vi "ALL2.vi"() -> ()   [LabVIEW 2016, in "Test2.lvrbt"]
uses:
  Test2.lvrbt
  <vilib>/NXT/Hardware/Plugins/Tetrix DC Motor/TetrixDCMotorAddress.ctl
  <vilib>/NXT/Hardware/Plugins/Tetrix 180 deg Servo/Tetrix180ServoAddress.ctl
  <vilib>/NXT/Block Support/NXT_InputPort.ctl
  <vilib>/NXT/Subs/ColorSensorColors.ctl
  <vilib>/NXT/NXTIO Xnodes/NXTIONodeSubVIs/TETRIX IO Move Servos.vi
  <vilib>/NXT/Dual Mode Library/Waits/Wait_Num.vi
  <vilib>/NXT/NXTIO Xnodes/NXTIONodeSubVIs/TETRIX IO Move DC Motors.vi
  <vilib>/NXT/NXTIO Xnodes/NXTIONodeSubVIs/TETRIX IO Stop DC Motors.vi
  <vilib>/NXT/Dual Mode Library/Waits/Wait_EV3_Ultrasonic_Centimeter_Closer.vi
  <vilib>/NXT/Dual Mode Library/Waits/Wait_EV3_Ultrasonic_Centimeters_Further.vi
  <vilib>/NXT/Dual Mode Library/Waits/Wait_Touch.vi
  <vilib>/NXT/Dual Mode Library/Waits/Wait_EV3_Color_Color.vi
  <vilib>/NXT/Dual Mode Library/Sensors/EV3_Ultrasonic_CM.vi
  <vilib>/NXT/NXTIO Xnodes/AddressXNode/NXTIOAddress.xnode
  <vilib>/NXT/Subs/LVHSConnector.ctl
  <vilib>/NXT/NXTIO Xnodes/NXTIOXNode/NXTIO.xnode
  <vilib>/NXT/LegoClasses/BrickReference/BrickReference.lvclass
panel:
  out "Power 3":bool
  out "X Upper Left  2":u8
  out "X Lower Right  2":u8
  out "Y Lower Right  2":u8
  out "Y Upper Left  2":u8
  out "Count 3":u8
  out "Color 3":u8
  in  "Cluster 3":T1 {"Tracking Mode" items=["Disable Tracking", "Get First Object", "Get n th Object", "Enable Tracking", "Sort Objects  by size", "Sort Objects  by Colors", "Illumination on ", "Illumination Off", "Write Colormap", "Read Colormap", "Line tracking mode", "Object Tracking mode"]}
  out "Power 2":bool
  out "X Upper Left":u8
  out "X Lower Right":u8
  out "Y Lower Right":u8
  out "Y Upper Left":u8
  out "Count 2":u8
  out "Color 2":u8
  in  "Cluster 2":T1 {"Tracking Mode" items=["Disable Tracking", "Get First Object", "Get n th Object", "Enable Tracking", "Sort Objects  by size", "Sort Objects  by Colors", "Illumination on ", "Illumination Off", "Write Colormap", "Read Colormap", "Line tracking mode", "Object Tracking mode"]}
types:
  T1 = cluster{"Address":dbl, "No of Object to track":dbl, "Tracking Mode":u8}
  T2 = typedef "Tetrix180ServoAddress.ctl" = i32
  T3 = cluster{"Tetrix180Servo":T2, "Tetrix180Servo 2":T2, "Tetrix180Servo 3":T2, "Tetrix180Servo 4":T2, "Tetrix180Servo 5":T2, "Tetrix180Servo 6":T2}
  T4 = typedef "TetrixDCMotorAddress.ctl" = i32
  T5 = cluster{"TetrixDCMotor":T4, "TetrixDCMotor 2":T4}
  T6 = cluster{"Tetrix180Servo":T2, "Tetrix180Servo":T2, "Tetrix180Servo":T2, "Tetrix180Servo":T2, "Tetrix180Servo":T2, "Tetrix180Servo":T2}
  T7 = typedef "LVHSConnector.ctl" = refnum<class "BrickReference.lvclass">
  T8 = typedef "NXT_InputPort.ctl" = u32
  T9 = typedef "ColorSensorColors.ctl" = enum16{"No Color", "Black", "Blue", "Green", "Yellow", "Red", "White", "Brown"}
  T10 = cluster{"Tracking Mode":u8, "Object Number to Track":u8, "Address":u8}
  T11 = cluster{"Total Tracked Objects":u8, "Color":u8, "X Upper Left":u8, "Y Upper Left":u8, "X Lower Right":u8, "Y Lower Right":u8, "Status (boolean)":bool}
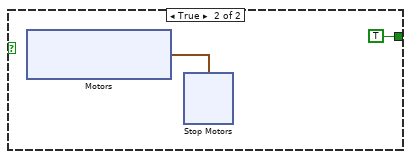
[diagram p2: hidden frame]
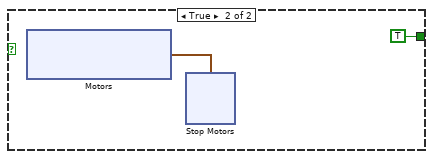
[diagram p3: hidden frame]
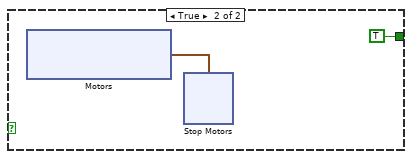
[diagram p4: hidden frame]
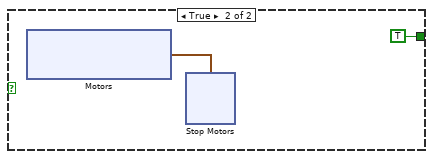
[diagram p5: hidden frame]
diagram:
  # "FILE: BACK TOBASE2\n\nTHE ROBOT WILL GO TO BASE"
  # "FILE: SAVETOUCH \n\nTHE ROBOT WILL DETECT THE RACK \nAND STRAIGHT THE POSITION"
  # "FILE: SAVETOUCH \n\nTHE ROBOT WILL DETECT THE RACK \nAND STRAIGHT THE POSITION"
  # "FILE: DETECT REFERENCE LINE, AFTER AIMING\n\nTHE ROBOT WILL GET A NEW POSITION AFTER LAUNCH THE BALL"
  # "FILE: TRAPBALL\n\nTHE ROBOT WILL MOVE FOWARD TO TRAP THE BALL"
  # "FILE: GETSEECONDBALL\n\nTHE ROBOT WILL START TO DETECT AND PICKUP THE SECOND BALL"
  # "FILE: DETECT REFERENCE LINE, AFTER AIMING\n\nTHE ROBOT WILL GET A NEW POSITION AFTER LAUNCH THE BALL"
  # "FILE: SERVOSETTING\n\nTHE FIRST BALL WILL BE PICKUP"
  # "FILE: DETECTFIRSTBALL\n\nTHE ROBOT WILL MOVE INFRONT TO DETECT THE FIRST BALL"
  # "FILE: SAVETOUCH \n\nTHE ROBOT WILL DETECT THE RACK \nAND STRAIGHT THE POSITION"
  # "FILE:  motor setting\n\nTHE ROBOT WILL MOVE OUT FROM THE BASE."
  n1 = flat-sequence {
    tunnel: [w13] -> w12
    frame #0 {
      n2 = xnode "Motors"() -> ("Motor"=w22:T6)
      n3 = xnode "Move Servos"("Position 6"=u8 28, "Position 5"=u8 237, "Position 4"=u8 40, "Position 3"=u8 7, "Position 2"=u8 0, "Position 1"=u8 220, "Motors"=w22) -> ("NXT/EV3"=w15:T7)  [unwired: 1 in]
      n4 = xnode "Motors"() -> ("Motor"=w27:cluster{"TetrixDCMotor":T4, "TetrixDCMotor":T4})
      n5 = call-poly <vilib>:"PolyWait.vi"("Time (1 sec)"=sgl 1.0, "NXT/EV3"=w15) -> ("NXT/EV3"=w14:T7)  [unwired: 2 in]
      n6 = xnode "Move Motors"("Power/Speed 2"=i8 50, "Power/Speed 1"=i8 50, "Motors"=w27, "NXT/EV3"=w14) -> ("NXT/EV3"=w30:T7)
      n7 = call-poly <vilib>:"PolyWait.vi"("Time (1 sec)"=sgl 2.0, "NXT/EV3"=w30) -> ("NXT/EV3"=w28:T7)  [unwired: 2 in]
      n8 = xnode "Motors"() -> ("Motor"=w33:cluster{"TetrixDCMotor":T4, "TetrixDCMotor":T4})
      n9 = xnode "Stop Motors"("Motors"=w27, "NXT/EV3"=w28) -> ("NXT/EV3"=w26:T7)
      n10 = call-poly <vilib>:"PolyWait.vi"("Time (1 sec)"=sgl 1.0, "NXT/EV3"=w26) -> ("NXT/EV3"=w24:T7)  [unwired: 2 in]
      n11 = xnode "Move Motors"("Power/Speed 2"=i8 50, "Power/Speed 1"=i8 50, "Motors"=w33, "NXT/EV3"=w24) -> ("NXT/EV3"=w36:T7)
      n12 = call-poly <vilib>:"PolyWait.vi"("Time (1 sec)"=sgl 1.5, "NXT/EV3"=w36) -> ("NXT/EV3"=w34:T7)  [unwired: 2 in]
      n13 = xnode "Stop Motors"("Motors"=w33, "NXT/EV3"=w34) -> ("NXT/EV3"=w13:T7)
    }
  }
  n14 = flat-sequence {
    tunnel: w12 -> [w82]
    tunnel: [w81] -> w11
    frame #0 {
      w97 = T8 1 items=["Port 1", "Port 2", "Port 3", "Port 4"] ("Port (Port 1)")
      w113 = T8 1 items=["Port 1", "Port 2", "Port 3", "Port 4"] ("Port (Port 1)")
      n15 = xnode "Motors"() -> ("Motor"=w126:cluster{"TetrixDCMotor":T4, "TetrixDCMotor":T4})
      n16 = call-poly <vilib>:"PolyWait.vi"("Time (1 sec)"=sgl 1.0, "NXT/EV3"=w82) -> ("NXT/EV3"=w83:T7)  [unwired: 2 in]
      n17 = xnode "Move Motors"("Power/Speed 2"=i8 50, "Power/Speed 1"=i8 50, "Motors"=w126, "NXT/EV3"=w83) -> ("NXT/EV3"=w129:T7)
      n18 = call-poly <vilib>:"PolyWait.vi"("Centimeters (40)"=sgl 8.0, "NXT/EV3"=w129, "Port (Port 1)"=w113) -> ("NXT/EV3"=w127:T7)  [unwired: 1 in]
      n19 = xnode "Motors"() -> ("Motor"=w94:cluster{"TetrixDCMotor":T4, "TetrixDCMotor":T4})
      n20 = xnode "Stop Motors"("Motors"=w126, "NXT/EV3"=w127) -> ("NXT/EV3"=w103:T7)
      n21 = call-poly <vilib>:"PolyWait.vi"("Time (1 sec)"=sgl 1.0, "NXT/EV3"=w103) -> ("NXT/EV3"=w86:T7)  [unwired: 2 in]
      n22 = xnode "Move Motors"("Power/Speed 2"=i8 -5, "Power/Speed 1"=i8 -5, "Motors"=w94, "NXT/EV3"=w86) -> ("NXT/EV3"=w100:T7)
      n23 = call-poly <vilib>:"PolyWait.vi"("Centimeters (50)"=sgl 6.0, "NXT/EV3"=w100, "Port (Port 1)"=w97) -> ("NXT/EV3"=w98:T7)  [unwired: 1 in]
      n24 = xnode "Motors"() -> ("Motor"=w88:cluster{"TetrixDCMotor":T4, "TetrixDCMotor":T4})
      n25 = xnode "Stop Motors"("Motors"=w94, "NXT/EV3"=w98) -> ("NXT/EV3"=w92:T7)
      n26 = call-poly <vilib>:"PolyWait.vi"("Time (1 sec)"=sgl 1.0, "NXT/EV3"=w92) -> ("NXT/EV3"=w91:T7)  [unwired: 2 in]
      n27 = xnode "Move Motors"("Power/Speed 2"=i8 5, "Power/Speed 1"=i8 5, "Motors"=w88, "NXT/EV3"=w91) -> ("NXT/EV3"=w90:T7)
      n28 = call-poly <vilib>:"PolyWait.vi"("Time (1 sec)"=sgl 1.0, "NXT/EV3"=w90) -> ("NXT/EV3"=w89:T7)  [unwired: 2 in]
      n29 = xnode "Motors"() -> ("Motor"=w122:T4)
      n30 = xnode "Motors"() -> ("Motor"=w118:T4)
      n31 = xnode "Stop Motors"("Motors"=w88, "NXT/EV3"=w89) -> ("NXT/EV3"=w85:T7)
      n32 = call-poly <vilib>:"PolyWait.vi"("Time (1 sec)"=sgl 1.5, "NXT/EV3"=w85) -> ("NXT/EV3"=w116:T7)  [unwired: 2 in]
      n33 = xnode "Motors"() -> ("Sensor"=w115:T8)
      n34 = xnode "Motors"() -> ("Sensor"=w114:T8)
      n35 = xnode "Move Motors"("Power/Speed 1"=i8 20, "Motors"=w122, "NXT/EV3"=w116) -> ("NXT/EV3"=w124:T7)
      n36 = xnode "Move Motors"("Power/Speed 1"=i8 20, "Motors"=w118, "NXT/EV3"=w116) -> ("NXT/EV3"=w119:T7)
      n37 = call-poly <vilib>:"PolyWait.vi"("NXT/EV3"=w124, "Port (Port 1)"=w114) -> ("NXT/EV3"=w123:T7)  [unwired: 2 in]
      n38 = call-poly <vilib>:"PolyWait.vi"("NXT/EV3"=w119, "Port (Port 1)"=w115) -> ("NXT/EV3"=w117:T7)  [unwired: 2 in]
      n39 = xnode "Motors"() -> ("Motor"=w80:cluster{"TetrixDCMotor":T4, "TetrixDCMotor":T4})
      n40 = xnode "Stop Motors"("Motors"=w122, "NXT/EV3"=w123) -> ()  [unwired: 1 out]
      n41 = xnode "Stop Motors"("Motors"=w118, "NXT/EV3"=w117) -> ("NXT/EV3"=w112:T7)
      n42 = call-poly <vilib>:"PolyWait.vi"("Time (1 sec)"=sgl 2.0, "NXT/EV3"=w112) -> ("NXT/EV3"=w109:T7)  [unwired: 2 in]
      n43 = xnode "Move Motors"("Power/Speed 2"=i8 -5, "Power/Speed 1"=i8 -5, "Motors"=w80, "NXT/EV3"=w109) -> ("NXT/EV3"=w106:T7)
      n44 = call-poly <vilib>:"PolyWait.vi"("Time (1 sec)"=sgl 0.2, "NXT/EV3"=w106) -> ("NXT/EV3"=w105:T7)  [unwired: 2 in]
      n45 = xnode "Stop Motors"("Motors"=w80, "NXT/EV3"=w105) -> ("NXT/EV3"=w81:T7)
    }
  }
  n46 = flat-sequence {
    tunnel: w11 -> [w217]
    tunnel: [w216] -> w10
    frame #0 {
      w232 = T8 1 items=["Port 1", "Port 2", "Port 3", "Port 4"] ("Port (Port 1)")
      n47 = xnode "Motors"() -> ("Motor"=w228:cluster{"TetrixDCMotor":T4, "TetrixDCMotor":T4})
      n48 = call-poly <vilib>:"PolyWait.vi"("Time (1 sec)"=sgl 1.0, "NXT/EV3"=w217) -> ("NXT/EV3"=w229:T7)  [unwired: 2 in]
      n49 = xnode "Move Motors"("Power/Speed 2"=i8 20, "Power/Speed 1"=i8 20, "Motors"=w228, "NXT/EV3"=w229) -> ("NXT/EV3"=w235:T7)
      n50 = call-poly <vilib>:"PolyWait.vi"("Centimeters (50)"=sgl 6.0, "NXT/EV3"=w235, "Port (Port 1)"=w232) -> ("NXT/EV3"=w233:T7)  [unwired: 1 in]
      n51 = xnode "Motors"() -> ("Motor"=w224:cluster{"TetrixDCMotor":T4, "TetrixDCMotor":T4})
      n52 = xnode "Stop Motors"("Motors"=w228, "NXT/EV3"=w233) -> ("NXT/EV3"=w218:T7)
      n53 = call-poly <vilib>:"PolyWait.vi"("Time (1 sec)"=sgl 1.0, "NXT/EV3"=w218) -> ("NXT/EV3"=w219:T7)  [unwired: 2 in]
      n54 = xnode "Motors"() -> ("Sensor"=w221:T8)
      n55 = xnode "Move Motors"("Power/Speed 2"=i8 -5, "Power/Speed 1"=i8 -5, "Motors"=w224, "NXT/EV3"=w219) -> ("NXT/EV3"=w226:T7)
      n56 = call-poly <vilib>:"PolyWait.vi"("Centimeters (40)"=sgl 11.0 ("Centimeters (50)"), "NXT/EV3"=w226, "Port (Port 1)"=w221) -> ("NXT/EV3"=w225:T7)  [unwired: 1 in]
      n57 = xnode "Stop Motors"("Motors"=w224, "NXT/EV3"=w225) -> ("NXT/EV3"=w216:T7)
    }
  }
  n58 = flat-sequence {
    tunnel: w10 -> [w267]
    tunnel: [w266] -> w9
    frame #0 {
      n59 = xnode "Motors"() -> ("Motor"=w272:T2)
      n60 = call-poly <vilib>:"PolyWait.vi"("Time (1 sec)"=sgl 1.0, "NXT/EV3"=w267) -> ("NXT/EV3"=w269:T7)  [unwired: 2 in]
      n61 = xnode "Move Servos"("Position 1"=u8 144, "Motors"=w272, "NXT/EV3"=w269) -> ("NXT/EV3"=w270:T7)
      n62 = xnode "Motors"() -> ("Motor"=w301:T2)
      n63 = call-poly <vilib>:"PolyWait.vi"("Time (1 sec)"=sgl 1.0, "NXT/EV3"=w270) -> ("NXT/EV3"=w283:T7)  [unwired: 2 in]
      n64 = xnode "Move Servos"("Position 1"=u8 70, "Motors"=w301, "NXT/EV3"=w283) -> ("NXT/EV3"=w298:T7)
      n65 = xnode "Motors"() -> ("Motor"=w297:T2)
      n66 = call-poly <vilib>:"PolyWait.vi"("Time (1 sec)"=sgl 7.0, "NXT/EV3"=w298) -> ("NXT/EV3"=w295:T7)  [unwired: 2 in]
      n67 = xnode "Move Servos"("Position 1"=u8 227, "Motors"=w297, "NXT/EV3"=w295) -> ("NXT/EV3"=w293:T7)
      n68 = xnode "Motors"() -> ("Motor"=w292:T2)
      n69 = call-poly <vilib>:"PolyWait.vi"("Time (1 sec)"=sgl 0.5, "NXT/EV3"=w293) -> ("NXT/EV3"=w290:T7)  [unwired: 2 in]
      n70 = xnode "Move Servos"("Position 1"=u8 8, "Motors"=w292, "NXT/EV3"=w290) -> ("NXT/EV3"=w288:T7)
      n71 = xnode "Motors"() -> ("Motor"=w286:T2)
      n72 = call-poly <vilib>:"PolyWait.vi"("Time (1 sec)"=sgl 1.0, "NXT/EV3"=w288) -> ("NXT/EV3"=w285:T7)  [unwired: 2 in]
      n73 = xnode "Move Servos"("Position 1"=u8 82, "Motors"=w286, "NXT/EV3"=w285) -> ("NXT/EV3"=w268:T7)
      n74 = xnode "Motors"() -> ("Motor"=w280:T2)
      n75 = call-poly <vilib>:"PolyWait.vi"("Time (1 sec)"=sgl 1.0, "NXT/EV3"=w268) -> ("NXT/EV3"=w279:T7)  [unwired: 2 in]
      n76 = xnode "Move Servos"("Position 1"=u8 67, "Motors"=w280, "NXT/EV3"=w279) -> ("NXT/EV3"=w277:T7)
      n77 = xnode "Motors"() -> ("Motor"=w275:T2)
      n78 = call-poly <vilib>:"PolyWait.vi"("Time (1 sec)"=sgl 1.0, "NXT/EV3"=w277) -> ("NXT/EV3"=w274:T7)  [unwired: 2 in]
      n79 = xnode "Move Servos"("Position 1"=u8 240, "Motors"=w275, "NXT/EV3"=w274) -> ("NXT/EV3"=w266:T7)
    }
  }
  n80 = flat-sequence {
    tunnel: w9 -> [w381]
    tunnel: [w380] -> w8
    frame #0 {
      w368 = T8 2 items=["Port 1", "Port 2", "Port 3", "Port 4"] ("Port (Port 1)")
      w366 = T8 3 items=["Port 1", "Port 2", "Port 3", "Port 4"] ("Input Port")
      # "FILE: LAUNCHFIRSTBALL\n\nTHE FIRST BALL WILL BE  LAUNCH"
      n81 = xnode "Motors"() -> ("Motor"=w415:T2)
      n82 = call-poly <vilib>:"PolyWait.vi"("Time (1 sec)"=sgl 1.0, "NXT/EV3"=w381) -> ("NXT/EV3"=w382:T7)  [unwired: 2 in]
      n83 = xnode "Move Servos"("Position 1"=u8 255, "Motors"=w415, "NXT/EV3"=w382) -> ("NXT/EV3"=w412:T7)
      n84 = xnode "Motors"() -> ("Motor"=w416:cluster{"TetrixDCMotor":T4, "TetrixDCMotor":T4})
      n85 = call-poly <vilib>:"PolyWait.vi"("Time (1 sec)"=sgl 1.0, "NXT/EV3"=w412) -> ("NXT/EV3"=w411:T7)  [unwired: 2 in]
      n86 = xnode "Move Motors"("Power/Speed 2"=i8 -50, "Power/Speed 1"=i8 -50, "Motors"=w416, "NXT/EV3"=w411) -> ("NXT/EV3"=w419:T7)
      n87 = call-poly <vilib>:"PolyWait.vi"("Time (1 sec)"=sgl 1.0, "NXT/EV3"=w419) -> ("NXT/EV3"=w417:T7)  [unwired: 2 in]
      n88 = xnode "Motors"() -> ("Motor"=w408:T2)
      n89 = xnode "Stop Motors"("Motors"=w416, "NXT/EV3"=w417) -> ("NXT/EV3"=w379:T7)
      n90 = call-poly <vilib>:"PolyWait.vi"("Time (1 sec)"=sgl 1.0, "NXT/EV3"=w379) -> ("NXT/EV3"=w409:T7)  [unwired: 2 in]
      n91 = xnode "Move Servos"("Position 1"=u8 0, "Motors"=w408, "NXT/EV3"=w409) -> ("NXT/EV3"=w402:T7)
      n92 = xnode "Motors"() -> ("Motor"=w404:T2)
      n93 = call-poly <vilib>:"PolyWait.vi"("Time (1 sec)"=sgl 1.0, "NXT/EV3"=w402) -> ("NXT/EV3"=w405:T7)  [unwired: 2 in]
      n94 = xnode "Move Servos"("Position 1"=u8 230, "Motors"=w404, "NXT/EV3"=w405) -> ("NXT/EV3"=w397:T7)
      n95 = xnode "Motors"() -> ("Motor"=w399:T2)
      n96 = call-poly <vilib>:"PolyWait.vi"("Time (1 sec)"=sgl 1.0, "NXT/EV3"=w397) -> ("NXT/EV3"=w400:T7)  [unwired: 2 in]
      n97 = xnode "Move Servos"("Position 1"=u8 7, "Motors"=w399, "NXT/EV3"=w400) -> ("NXT/EV3"=w392:T7)
      n98 = xnode "Motors"() -> ("Motor"=w394:T2)
      n99 = call-poly <vilib>:"PolyWait.vi"("Time (1 sec)"=sgl 0.5, "NXT/EV3"=w392) -> ("NXT/EV3"=w395:T7)  [unwired: 2 in]
      n100 = xnode "Move Servos"("Position 1"=u8 220, "Motors"=w394, "NXT/EV3"=w395) -> ("NXT/EV3"=w360:T7)
      n101 = xnode "Motors"() -> ("Motor"=w375:cluster{"TetrixDCMotor":T4, "TetrixDCMotor":T4})
      n102 = call-poly <vilib>:"PolyWait.vi"("Time (1 sec)"=sgl 1.0, "NXT/EV3"=w360) -> ("NXT/EV3"=w358:T7)  [unwired: 2 in]
      n103 = xnode "Move Motors"("Power/Speed 2"=i8 50, "Power/Speed 1"=i8 50, "Motors"=w375, "NXT/EV3"=w358) -> ("NXT/EV3"=w370:T7)
      n104 = call-poly <vilib>:"PolyWait.vi"("Color (Red)"=ColorSensorColors."Black", "NXT/EV3"=w370, "Port (Port 1)"=w368) -> ("NXT/EV3"=w369:T7)  [unwired: 1 in]
      n105 = xnode "Stop Motors"("Motors"=w375, "NXT/EV3"=w369) -> ("NXT/EV3"=w374:T7)
      n106 = call-poly <vilib>:"PolyWait.vi"("Time (1 sec)"=sgl 1.0, "NXT/EV3"=w374) -> ("NXT/EV3"=w373:T7)  [unwired: 2 in]
      n107 = call "NXTCam-DM.vi"("Input of NXTCam"=T10 {"Tracking Mode"=3, "Object Number to Track"=1, "Address"=1}, "NXT"=w373, "Input Port"=w366) -> ("NXT dup"=w367:T7)  [unwired: 1 out]
      n108 = while {
        tunnel: w367 -> [w463]
        tunnel: w366 -> [w462]
        tunnel: [w460] -> w364
        stop <- w461 stop-if-true
        n109 = call "NXTCam-DM.vi"("Input of NXTCam"="Cluster 2", "NXT"=w463, "Input Port"=w462) -> ("Output of NXTCam"=w470:T11, "NXT dup"=w460:T7)
        n110 = Unbundle By Name(w470) -> ("Total Tracked Objects"=→"Count 2":u8, "Color"=→"Color 2":u8, "X Upper Left"=w459:u8, "Y Upper Left"=→"Y Upper Left":u8, "X Lower Right"=w467:u8, "Y Lower Right"=→"Y Lower Right":u8, "Status (boolean)"=→"Power 2":bool)
        "X Upper Left" <- w459
        "X Lower Right" <- w467
        n111 = xnode "Motors"() -> ("Sensor"=w453:T8)
        n112 = call-poly <vilib>:"PolySensor.vi"("Port (Port 1)"=w453) -> ("Centimeters"=w455:sgl)  [unwired: 2 in, 1 out]
        n113 = Greater?(x=w459, y=u8 41) -> (0:w465:bool)
        n114 = Less?(x=w467, y=u8 100) -> (x < y?=w464:bool)
        n115 = And(x=w465, y=w464) -> (x .and. y?=w457:bool)
        n116 = Greater?(x=w455, y=sgl 5.5) -> (0:w454:bool)
        n117 = Or(x=w457, y=w454) -> (x .or. y?=w456:bool)
        n118 = case shown="False" w456 {
          tunnel: [FALSE TRUE] -> w461
          frame False {
            n119 = xnode "Motors"() -> ("Motor"=w480:cluster{"TetrixDCMotor":T4, "TetrixDCMotor":T4})
            n120 = xnode "Move Motors"("Power/Speed 2"=i8 -18, "Power/Speed 1"=i8 -10, "Motors"=w480) -> ()  [unwired: 1 in, 1 out]
          }
          frame True {
            n121 = xnode "Motors"() -> ("Motor"=w491:cluster{"TetrixDCMotor":T4, "TetrixDCMotor":T4})
            n122 = xnode "Stop Motors"("Motors"=w491) -> ()  [unwired: 1 in, 1 out]
          }
        }
      }
      n123 = call-poly <vilib>:"PolyWait.vi"("Time (1 sec)"=sgl 1.0, "NXT/EV3"=w364) -> ("NXT/EV3"=w363:T7)  [unwired: 2 in]
      n124 = while {
        tunnel: w363 -> [w428]
        tunnel: [w423] -> w361
        stop <- w425 stop-if-true
        n125 = xnode "Motors"() -> ("Sensor"=w422:T8)
        n126 = call-poly <vilib>:"PolySensor.vi"("NXT/EV3"=w428, "Port (Port 1)"=w422) -> ("Centimeters"=w427:sgl, "NXT/EV3"=w423:T7)  [unwired: 1 in]
        n127 = Less?(x=w427, y=sgl 5.5) -> (x < y?=w424:bool)
        n128 = case shown="False" w424 {
          tunnel: [FALSE TRUE] -> w425
          frame False {
            n129 = xnode "Motors"() -> ("Motor"=w435:cluster{"TetrixDCMotor":T4, "TetrixDCMotor":T4})
            n130 = xnode "Move Motors"("Power/Speed 2"=i8 20, "Power/Speed 1"=i8 20, "Motors"=w435) -> ("NXT/EV3"=w432:T7)  [unwired: 1 in]
            n131 = call-poly <vilib>:"PolyWait.vi"("Time (1 sec)"=sgl 1.5, "NXT/EV3"=w432) -> ()  [unwired: 2 in, 1 out]
          }
          frame True {
            n132 = xnode "Motors"() -> ("Motor"=w446:cluster{"TetrixDCMotor":T4, "TetrixDCMotor":T4})
            n133 = xnode "Stop Motors"("Motors"=w446) -> ()  [unwired: 1 in, 1 out]
          }
        }
      }
      n134 = xnode "Motors"() -> ("Motor"=w390:T2)
      n135 = call-poly <vilib>:"PolyWait.vi"("Time (1 sec)"=sgl 0.8, "NXT/EV3"=w361) -> ("NXT/EV3"=w359:T7)  [unwired: 2 in]
      n136 = xnode "Move Servos"("Position 1"=u8 114, "Motors"=w390, "NXT/EV3"=w359) -> ("NXT/EV3"=w384:T7)
      n137 = xnode "Motors"() -> ("Motor"=w386:T2)
      n138 = call-poly <vilib>:"PolyWait.vi"("Time (1 sec)"=sgl 1.5, "NXT/EV3"=w384) -> ("NXT/EV3"=w387:T7)  [unwired: 2 in]
      n139 = xnode "Move Servos"("Position 1"=u8 40, "Motors"=w386, "NXT/EV3"=w387) -> ("NXT/EV3"=w380:T7)
    }
  }
  n140 = flat-sequence {
    tunnel: w8 -> [w593]
    tunnel: [w582] -> w7
    frame #0 {
      w596 = T8 2 items=["Port 1", "Port 2", "Port 3", "Port 4"] ("Port (Port 1)")
      w605 = T8 2 items=["Port 1", "Port 2", "Port 3", "Port 4"] ("Port (Port 1)")
      n141 = xnode "Motors"() -> ("Motor"=w615:cluster{"TetrixDCMotor":T4, "TetrixDCMotor":T4})
      n142 = call-poly <vilib>:"PolyWait.vi"("Time (1 sec)"=sgl 1.0, "NXT/EV3"=w593) -> ("NXT/EV3"=w592:T7)  [unwired: 2 in]
      n143 = xnode "Move Motors"("Power/Speed 2"=i8 -50, "Power/Speed 1"=i8 -50, "Motors"=w615, "NXT/EV3"=w592) -> ("NXT/EV3"=w618:T7)
      n144 = call-poly <vilib>:"PolyWait.vi"("Time (1 sec)"=sgl 0.8, "NXT/EV3"=w618) -> ("NXT/EV3"=w617:T7)  [unwired: 2 in]
      n145 = xnode "Motors"() -> ("Motor"=w610:cluster{"TetrixDCMotor":T4, "TetrixDCMotor":T4})
      n146 = xnode "Stop Motors"("Motors"=w615, "NXT/EV3"=w617) -> ("NXT/EV3"=w608:T7)
      n147 = call-poly <vilib>:"PolyWait.vi"("Time (1 sec)"=sgl 1.0, "NXT/EV3"=w608) -> ("NXT/EV3"=w607:T7)  [unwired: 2 in]
      n148 = xnode "Move Motors"("Power/Speed 2"=i8 20, "Power/Speed 1"=i8 20, "Motors"=w610, "NXT/EV3"=w607) -> ("NXT/EV3"=w612:T7)
      n149 = call-poly <vilib>:"PolyWait.vi"("Color (Red)"=ColorSensorColors."Black", "NXT/EV3"=w612, "Port (Port 1)"=w605) -> ("NXT/EV3"=w611:T7)  [unwired: 1 in]
      n150 = xnode "Motors"() -> ("Motor"=w600:cluster{"TetrixDCMotor":T4, "TetrixDCMotor":T4})
      n151 = xnode "Stop Motors"("Motors"=w610, "NXT/EV3"=w611) -> ("NXT/EV3"=w595:T7)
      n152 = call-poly <vilib>:"PolyWait.vi"("Time (1 sec)"=sgl 0.5, "NXT/EV3"=w595) -> ("NXT/EV3"=w598:T7)  [unwired: 2 in]
      n153 = xnode "Move Motors"("Power/Speed 2"=i8 -20, "Power/Speed 1"=i8 -20, "Motors"=w600, "NXT/EV3"=w598) -> ("NXT/EV3"=w602:T7)
      n154 = call-poly <vilib>:"PolyWait.vi"("Color (Red)"=ColorSensorColors."Black", "NXT/EV3"=w602, "Port (Port 1)"=w596) -> ("NXT/EV3"=w601:T7)  [unwired: 1 in]
      n155 = xnode "Motors"() -> ("Motor"=w586:cluster{"TetrixDCMotor":T4, "TetrixDCMotor":T4})
      n156 = xnode "Stop Motors"("Motors"=w600, "NXT/EV3"=w601) -> ("NXT/EV3"=w584:T7)
      n157 = call-poly <vilib>:"PolyWait.vi"("Time (1 sec)"=sgl 0.5, "NXT/EV3"=w584) -> ("NXT/EV3"=w583:T7)  [unwired: 2 in]
      n158 = xnode "Move Motors"("Power/Speed 2"=i8 -5, "Power/Speed 1"=i8 -5, "Motors"=w586, "NXT/EV3"=w583) -> ("NXT/EV3"=w589:T7)
      n159 = call-poly <vilib>:"PolyWait.vi"("Time (1 sec)"=sgl 1.0, "NXT/EV3"=w589) -> ("NXT/EV3"=w588:T7)  [unwired: 2 in]
      n160 = xnode "Stop Motors"("Motors"=w586, "NXT/EV3"=w588) -> ("NXT/EV3"=w582:T7)
    }
  }
  n161 = flat-sequence {
    tunnel: w7 -> [w680]
    tunnel: [w678] -> w6
    frame #0 {
      w695 = T8 1 items=["Port 1", "Port 2", "Port 3", "Port 4"] ("Port (Port 1)")
      w722 = T8 1 items=["Port 1", "Port 2", "Port 3", "Port 4"] ("Port (Port 1)")
      n162 = xnode "Motors"() -> ("Motor"=w711:T6)
      n163 = call-poly <vilib>:"PolyWait.vi"("Time (1 sec)"=sgl 1.0, "NXT/EV3"=w680) -> ("NXT/EV3"=w681:T7)  [unwired: 2 in]
      n164 = xnode "Move Servos"("Position 6"=u8 28, "Position 5"=u8 237, "Position 4"=u8 40, "Position 3"=u8 7, "Position 2"=u8 0, "Position 1"=u8 220, "Motors"=w711, "NXT/EV3"=w681) -> ("NXT/EV3"=w704:T7)
      n165 = xnode "Motors"() -> ("Motor"=w735:cluster{"TetrixDCMotor":T4, "TetrixDCMotor":T4})
      n166 = call-poly <vilib>:"PolyWait.vi"("Time (1 sec)"=sgl 1.0, "NXT/EV3"=w704) -> ("NXT/EV3"=w703:T7)  [unwired: 2 in]
      n167 = xnode "Move Motors"("Power/Speed 2"=i8 50, "Power/Speed 1"=i8 50, "Motors"=w735, "NXT/EV3"=w703) -> ("NXT/EV3"=w738:T7)
      n168 = call-poly <vilib>:"PolyWait.vi"("Centimeters (40)"=sgl 8.0, "NXT/EV3"=w738, "Port (Port 1)"=w722) -> ("NXT/EV3"=w736:T7)  [unwired: 1 in]
      n169 = xnode "Motors"() -> ("Motor"=w692:cluster{"TetrixDCMotor":T4, "TetrixDCMotor":T4})
      n170 = xnode "Stop Motors"("Motors"=w735, "NXT/EV3"=w736) -> ("NXT/EV3"=w701:T7)
      n171 = call-poly <vilib>:"PolyWait.vi"("Time (1 sec)"=sgl 1.0, "NXT/EV3"=w701) -> ("NXT/EV3"=w684:T7)  [unwired: 2 in]
      n172 = xnode "Move Motors"("Power/Speed 2"=i8 -5, "Power/Speed 1"=i8 -5, "Motors"=w692, "NXT/EV3"=w684) -> ("NXT/EV3"=w698:T7)
      n173 = call-poly <vilib>:"PolyWait.vi"("Centimeters (50)"=sgl 6.0, "NXT/EV3"=w698, "Port (Port 1)"=w695) -> ("NXT/EV3"=w696:T7)  [unwired: 1 in]
      n174 = xnode "Motors"() -> ("Motor"=w686:cluster{"TetrixDCMotor":T4, "TetrixDCMotor":T4})
      n175 = xnode "Stop Motors"("Motors"=w692, "NXT/EV3"=w696) -> ("NXT/EV3"=w690:T7)
      n176 = call-poly <vilib>:"PolyWait.vi"("Time (1 sec)"=sgl 1.0, "NXT/EV3"=w690) -> ("NXT/EV3"=w689:T7)  [unwired: 2 in]
      n177 = xnode "Move Motors"("Power/Speed 2"=i8 5, "Power/Speed 1"=i8 5, "Motors"=w686, "NXT/EV3"=w689) -> ("NXT/EV3"=w688:T7)
      n178 = call-poly <vilib>:"PolyWait.vi"("Time (1 sec)"=sgl 1.0, "NXT/EV3"=w688) -> ("NXT/EV3"=w687:T7)  [unwired: 2 in]
      n179 = xnode "Motors"() -> ("Motor"=w731:T4)
      n180 = xnode "Motors"() -> ("Motor"=w727:T4)
      n181 = xnode "Stop Motors"("Motors"=w686, "NXT/EV3"=w687) -> ("NXT/EV3"=w683:T7)
      n182 = call-poly <vilib>:"PolyWait.vi"("Time (1 sec)"=sgl 1.5, "NXT/EV3"=w683) -> ("NXT/EV3"=w725:T7)  [unwired: 2 in]
      n183 = xnode "Motors"() -> ("Sensor"=w724:T8)
      n184 = xnode "Motors"() -> ("Sensor"=w723:T8)
      n185 = xnode "Move Motors"("Power/Speed 1"=i8 20, "Motors"=w731, "NXT/EV3"=w725) -> ("NXT/EV3"=w733:T7)
      n186 = xnode "Move Motors"("Power/Speed 1"=i8 20, "Motors"=w727, "NXT/EV3"=w725) -> ("NXT/EV3"=w728:T7)
      n187 = call-poly <vilib>:"PolyWait.vi"("NXT/EV3"=w733, "Port (Port 1)"=w723) -> ("NXT/EV3"=w732:T7)  [unwired: 2 in]
      n188 = call-poly <vilib>:"PolyWait.vi"("NXT/EV3"=w728, "Port (Port 1)"=w724) -> ("NXT/EV3"=w726:T7)  [unwired: 2 in]
      n189 = xnode "Motors"() -> ("Motor"=w719:cluster{"TetrixDCMotor":T4, "TetrixDCMotor":T4})
      n190 = xnode "Stop Motors"("Motors"=w731, "NXT/EV3"=w732) -> ()  [unwired: 1 out]
      n191 = xnode "Stop Motors"("Motors"=w727, "NXT/EV3"=w726) -> ("NXT/EV3"=w721:T7)
      n192 = call-poly <vilib>:"PolyWait.vi"("Time (1 sec)"=sgl 2.0, "NXT/EV3"=w721) -> ("NXT/EV3"=w717:T7)  [unwired: 2 in]
      n193 = xnode "Move Motors"("Power/Speed 2"=i8 -5, "Power/Speed 1"=i8 -5, "Motors"=w719, "NXT/EV3"=w717) -> ("NXT/EV3"=w714:T7)
      n194 = call-poly <vilib>:"PolyWait.vi"("Time (1 sec)"=sgl 0.2, "NXT/EV3"=w714) -> ("NXT/EV3"=w713:T7)  [unwired: 2 in]
      n195 = xnode "Stop Motors"("Motors"=w719, "NXT/EV3"=w713) -> ("NXT/EV3"=w677:T7)
      n196 = call-poly <vilib>:"PolyWait.vi"("Time (1 sec)"=sgl 1.0, "NXT/EV3"=w677) -> ("NXT/EV3"=w678:T7)  [unwired: 2 in]
    }
  }
  n197 = flat-sequence {
    tunnel: w6 -> [w839]
    tunnel: [w838] -> w5
    frame #0 {
      w887 = T8 1 items=["Port 1", "Port 2", "Port 3", "Port 4"] ("Port (Port 1)")
      n198 = xnode "Motors"() -> ("Motor"=w882:T6)
      n199 = xnode "Move Servos"("Position 6"=u8 28, "Position 5"=u8 237, "Position 4"=u8 40, "Position 3"=u8 7, "Position 2"=u8 0, "Position 1"=u8 220, "Motors"=w882, "NXT/EV3"=w839) -> ("NXT/EV3"=w875:T7)
      n200 = xnode "Motors"() -> ("Motor"=w883:cluster{"TetrixDCMotor":T4, "TetrixDCMotor":T4})
      n201 = call-poly <vilib>:"PolyWait.vi"("Time (1 sec)"=sgl 0.5, "NXT/EV3"=w875) -> ("NXT/EV3"=w884:T7)  [unwired: 2 in]
      n202 = xnode "Move Motors"("Power/Speed 2"=i8 20, "Power/Speed 1"=i8 20, "Motors"=w883, "NXT/EV3"=w884) -> ("NXT/EV3"=w890:T7)
      n203 = call-poly <vilib>:"PolyWait.vi"("Centimeters (50)"=sgl 6.0, "NXT/EV3"=w890, "Port (Port 1)"=w887) -> ("NXT/EV3"=w888:T7)  [unwired: 1 in]
      n204 = xnode "Motors"() -> ("Motor"=w870:cluster{"TetrixDCMotor":T4, "TetrixDCMotor":T4})
      n205 = xnode "Stop Motors"("Motors"=w883, "NXT/EV3"=w888) -> ("NXT/EV3"=w874:T7)
      n206 = call-poly <vilib>:"PolyWait.vi"("Time (1 sec)"=sgl 1.0, "NXT/EV3"=w874) -> ("NXT/EV3"=w865:T7)  [unwired: 2 in]
      n207 = xnode "Motors"() -> ("Sensor"=w867:T8)
      n208 = xnode "Move Motors"("Power/Speed 2"=i8 -5, "Power/Speed 1"=i8 -5, "Motors"=w870, "NXT/EV3"=w865) -> ("NXT/EV3"=w872:T7)
      n209 = call-poly <vilib>:"PolyWait.vi"("Centimeters (40)"=sgl 6.0 ("Centimeters (50)"), "NXT/EV3"=w872, "Port (Port 1)"=w867) -> ("NXT/EV3"=w871:T7)  [unwired: 1 in]
      n210 = xnode "Motors"() -> ("Motor"=w844:T2)
      n211 = xnode "Stop Motors"("Motors"=w870, "NXT/EV3"=w871) -> ("NXT/EV3"=w840:T7)
      n212 = call-poly <vilib>:"PolyWait.vi"("Time (1 sec)"=sgl 1.0, "NXT/EV3"=w840) -> ("NXT/EV3"=w841:T7)  [unwired: 2 in]
      n213 = xnode "Move Servos"("Position 1"=u8 144, "Motors"=w844, "NXT/EV3"=w841) -> ("NXT/EV3"=w842:T7)
      n214 = xnode "Motors"() -> ("Motor"=w864:T2)
      n215 = call-poly <vilib>:"PolyWait.vi"("Time (1 sec)"=sgl 1.0, "NXT/EV3"=w842) -> ("NXT/EV3"=w846:T7)  [unwired: 2 in]
      n216 = xnode "Move Servos"("Position 1"=u8 70, "Motors"=w864, "NXT/EV3"=w846) -> ("NXT/EV3"=w861:T7)
      n217 = xnode "Motors"() -> ("Motor"=w860:T2)
      n218 = call-poly <vilib>:"PolyWait.vi"("Time (1 sec)"=sgl 7.0, "NXT/EV3"=w861) -> ("NXT/EV3"=w858:T7)  [unwired: 2 in]
      n219 = xnode "Move Servos"("Position 1"=u8 227, "Motors"=w860, "NXT/EV3"=w858) -> ("NXT/EV3"=w856:T7)
      n220 = xnode "Motors"() -> ("Motor"=w855:T2)
      n221 = call-poly <vilib>:"PolyWait.vi"("Time (1 sec)"=sgl 0.5, "NXT/EV3"=w856) -> ("NXT/EV3"=w853:T7)  [unwired: 2 in]
      n222 = xnode "Move Servos"("Position 1"=u8 8, "Motors"=w855, "NXT/EV3"=w853) -> ("NXT/EV3"=w851:T7)
      n223 = xnode "Motors"() -> ("Motor"=w849:T2)
      n224 = call-poly <vilib>:"PolyWait.vi"("Time (1 sec)"=sgl 1.0, "NXT/EV3"=w851) -> ("NXT/EV3"=w848:T7)  [unwired: 2 in]
      n225 = xnode "Move Servos"("Position 1"=u8 82, "Motors"=w849, "NXT/EV3"=w848) -> ("NXT/EV3"=w838:T7)
    }
  }
  n226 = flat-sequence {
    tunnel: w5 -> [w975]
    tunnel: [w974] -> w4
    frame #0 {
      w991 = T8 1 items=["Port 1", "Port 2", "Port 3", "Port 4"] ("Port (Port 1)")
      n227 = xnode "Motors"() -> ("Motor"=w988:cluster{"TetrixDCMotor":T4, "TetrixDCMotor":T4})
      n228 = call-poly <vilib>:"PolyWait.vi"("Time (1 sec)"=sgl 1.0, "NXT/EV3"=w975) -> ("NXT/EV3"=w986:T7)  [unwired: 2 in]
      n229 = xnode "Move Motors"("Power/Speed 1"=i8 20, "Motors"=w988, "NXT/EV3"=w986, "Power/Speed 2"=i8 20) -> ("NXT/EV3"=w994:T7)
      n230 = call-poly <vilib>:"PolyWait.vi"("Centimeters (50)"=sgl 6.0, "NXT/EV3"=w994, "Port (Port 1)"=w991) -> ("NXT/EV3"=w992:T7)  [unwired: 1 in]
      n231 = xnode "Motors"() -> ("Motor"=w983:T2)
      n232 = xnode "Stop Motors"("Motors"=w988, "NXT/EV3"=w992) -> ("NXT/EV3"=w976:T7)
      n233 = call-poly <vilib>:"PolyWait.vi"("Time (1 sec)"=sgl 1.0, "NXT/EV3"=w976) -> ("NXT/EV3"=w982:T7)  [unwired: 2 in]
      n234 = xnode "Move Servos"("Position 1"=u8 67, "Motors"=w983, "NXT/EV3"=w982) -> ("NXT/EV3"=w980:T7)
      n235 = xnode "Motors"() -> ("Motor"=w978:T2)
      n236 = call-poly <vilib>:"PolyWait.vi"("Time (1 sec)"=sgl 1.0, "NXT/EV3"=w980) -> ("NXT/EV3"=w977:T7)  [unwired: 2 in]
      n237 = xnode "Move Servos"("Position 1"=u8 240, "Motors"=w978, "NXT/EV3"=w977) -> ("NXT/EV3"=w974:T7)
    }
  }
  n238 = flat-sequence {
    tunnel: [w1046] -> w3
    tunnel: w4 -> [w1045]
    frame #0 {
      w1034 = T8 2 items=["Port 1", "Port 2", "Port 3", "Port 4"] ("Port (Port 1)")
      w1032 = T8 3 items=["Port 1", "Port 2", "Port 3", "Port 4"] ("Input Port")
      # "FILE: LAUNCHFIRSTBALL\n\nTHE SECOND BALL WILL BE  LAUNCH"
      n239 = xnode "Motors"() -> ("Motor"=w1082:T2)
      n240 = call-poly <vilib>:"PolyWait.vi"("Time (1 sec)"=sgl 1.0, "NXT/EV3"=w1045) -> ("NXT/EV3"=w1047:T7)  [unwired: 2 in]
      n241 = xnode "Move Servos"("Position 1"=u8 255, "Motors"=w1082, "NXT/EV3"=w1047) -> ("NXT/EV3"=w1079:T7)
      n242 = xnode "Motors"() -> ("Motor"=w1083:cluster{"TetrixDCMotor":T4, "TetrixDCMotor":T4})
      n243 = call-poly <vilib>:"PolyWait.vi"("Time (1 sec)"=sgl 1.0, "NXT/EV3"=w1079) -> ("NXT/EV3"=w1078:T7)  [unwired: 2 in]
      n244 = xnode "Move Motors"("Power/Speed 2"=i8 -50, "Power/Speed 1"=i8 -50, "Motors"=w1083, "NXT/EV3"=w1078) -> ("NXT/EV3"=w1086:T7)
      n245 = call-poly <vilib>:"PolyWait.vi"("Time (1 sec)"=sgl 1.0, "NXT/EV3"=w1086) -> ("NXT/EV3"=w1084:T7)  [unwired: 2 in]
      n246 = xnode "Motors"() -> ("Motor"=w1074:T2)
      n247 = xnode "Stop Motors"("Motors"=w1083, "NXT/EV3"=w1084) -> ("NXT/EV3"=w1077:T7)
      n248 = call-poly <vilib>:"PolyWait.vi"("Time (1 sec)"=sgl 1.0, "NXT/EV3"=w1077) -> ("NXT/EV3"=w1075:T7)  [unwired: 2 in]
      n249 = xnode "Move Servos"("Position 1"=u8 0, "Motors"=w1074, "NXT/EV3"=w1075) -> ("NXT/EV3"=w1068:T7)
      n250 = xnode "Motors"() -> ("Motor"=w1070:T2)
      n251 = call-poly <vilib>:"PolyWait.vi"("Time (1 sec)"=sgl 1.0, "NXT/EV3"=w1068) -> ("NXT/EV3"=w1071:T7)  [unwired: 2 in]
      n252 = xnode "Move Servos"("Position 1"=u8 230, "Motors"=w1070, "NXT/EV3"=w1071) -> ("NXT/EV3"=w1063:T7)
      n253 = xnode "Motors"() -> ("Motor"=w1065:T2)
      n254 = call-poly <vilib>:"PolyWait.vi"("Time (1 sec)"=sgl 1.0, "NXT/EV3"=w1063) -> ("NXT/EV3"=w1066:T7)  [unwired: 2 in]
      n255 = xnode "Move Servos"("Position 1"=u8 7, "Motors"=w1065, "NXT/EV3"=w1066) -> ("NXT/EV3"=w1058:T7)
      n256 = xnode "Motors"() -> ("Motor"=w1060:T2)
      n257 = call-poly <vilib>:"PolyWait.vi"("Time (1 sec)"=sgl 0.5, "NXT/EV3"=w1058) -> ("NXT/EV3"=w1061:T7)  [unwired: 2 in]
      n258 = xnode "Move Servos"("Position 1"=u8 220, "Motors"=w1060, "NXT/EV3"=w1061) -> ("NXT/EV3"=w1054:T7)
      n259 = xnode "Motors"() -> ("Motor"=w1041:cluster{"TetrixDCMotor":T4, "TetrixDCMotor":T4})
      n260 = call-poly <vilib>:"PolyWait.vi"("Time (1 sec)"=sgl 1.0, "NXT/EV3"=w1054) -> ("NXT/EV3"=w1026:T7)  [unwired: 2 in]
      n261 = xnode "Move Motors"("Power/Speed 2"=i8 50, "Power/Speed 1"=i8 50, "Motors"=w1041, "NXT/EV3"=w1026) -> ("NXT/EV3"=w1036:T7)
      n262 = call-poly <vilib>:"PolyWait.vi"("Color (Red)"=ColorSensorColors."Black", "NXT/EV3"=w1036, "Port (Port 1)"=w1034) -> ("NXT/EV3"=w1035:T7)  [unwired: 1 in]
      n263 = xnode "Stop Motors"("Motors"=w1041, "NXT/EV3"=w1035) -> ("NXT/EV3"=w1040:T7)
      n264 = call-poly <vilib>:"PolyWait.vi"("Time (1 sec)"=sgl 1.0, "NXT/EV3"=w1040) -> ("NXT/EV3"=w1039:T7)  [unwired: 2 in]
      n265 = call "NXTCam-DM.vi"("Input of NXTCam"=T10 {"Tracking Mode"=3, "Object Number to Track"=1, "Address"=1}, "NXT"=w1039, "Input Port"=w1032) -> ("NXT dup"=w1033:T7)  [unwired: 1 out]
      n266 = while {
        tunnel: w1033 -> [w1130]
        tunnel: w1032 -> [w1129]
        tunnel: [w1127] -> w1030
        stop <- w1128 stop-if-true
        n267 = call "NXTCam-DM.vi"("Input of NXTCam"="Cluster 3", "NXT"=w1130, "Input Port"=w1129) -> ("Output of NXTCam"=w1137:T11, "NXT dup"=w1127:T7)
        n268 = Unbundle By Name(w1137) -> ("Total Tracked Objects"=→"Count 3":u8, "Color"=→"Color 3":u8, "X Upper Left"=w1126:u8, "Y Upper Left"=→"Y Upper Left  2":u8, "X Lower Right"=w1134:u8, "Y Lower Right"=→"Y Lower Right  2":u8, "Status (boolean)"=→"Power 3":bool)
        "X Upper Left  2" <- w1126
        "X Lower Right  2" <- w1134
        n269 = xnode "Motors"() -> ("Sensor"=w1120:T8)
        n270 = call-poly <vilib>:"PolySensor.vi"("Port (Port 1)"=w1120) -> ("Centimeters"=w1122:sgl)  [unwired: 2 in, 1 out]
        n271 = Greater?(x=w1126, y=u8 41) -> (0:w1132:bool)
        n272 = Less?(x=w1134, y=u8 100) -> (x < y?=w1131:bool)
        n273 = And(x=w1132, y=w1131) -> (x .and. y?=w1124:bool)
        n274 = Greater?(x=w1122, y=sgl 5.5) -> (0:w1121:bool)
        n275 = Or(x=w1124, y=w1121) -> (x .or. y?=w1123:bool)
        n276 = case shown="False" w1123 {
          tunnel: [FALSE TRUE] -> w1128
          frame False {
            n277 = xnode "Motors"() -> ("Motor"=w1147:cluster{"TetrixDCMotor":T4, "TetrixDCMotor":T4})
            n278 = xnode "Move Motors"("Power/Speed 2"=i8 -18, "Power/Speed 1"=i8 -10, "Motors"=w1147) -> ()  [unwired: 1 in, 1 out]
          }
          frame True {
            n279 = xnode "Motors"() -> ("Motor"=w1158:cluster{"TetrixDCMotor":T4, "TetrixDCMotor":T4})
            n280 = xnode "Stop Motors"("Motors"=w1158) -> ()  [unwired: 1 in, 1 out]
          }
        }
      }
      n281 = call-poly <vilib>:"PolyWait.vi"("Time (1 sec)"=sgl 0.8, "NXT/EV3"=w1030) -> ("NXT/EV3"=w1029:T7)  [unwired: 2 in]
      n282 = while {
        tunnel: w1029 -> [w1095]
        tunnel: [w1090] -> w1027
        stop <- w1092 stop-if-true
        n283 = xnode "Motors"() -> ("Sensor"=w1089:T8)
        n284 = call-poly <vilib>:"PolySensor.vi"("NXT/EV3"=w1095, "Port (Port 1)"=w1089) -> ("Centimeters"=w1094:sgl, "NXT/EV3"=w1090:T7)  [unwired: 1 in]
        n285 = Less?(x=w1094, y=sgl 5.5) -> (x < y?=w1091:bool)
        n286 = case shown="False" w1091 {
          tunnel: [FALSE TRUE] -> w1092
          frame False {
            n287 = xnode "Motors"() -> ("Motor"=w1102:cluster{"TetrixDCMotor":T4, "TetrixDCMotor":T4})
            n288 = xnode "Move Motors"("Power/Speed 2"=i8 20, "Power/Speed 1"=i8 20, "Motors"=w1102) -> ("NXT/EV3"=w1099:T7)  [unwired: 1 in]
            n289 = call-poly <vilib>:"PolyWait.vi"("Time (1 sec)"=sgl 1.5, "NXT/EV3"=w1099) -> ()  [unwired: 2 in, 1 out]
          }
          frame True {
            n290 = xnode "Motors"() -> ("Motor"=w1113:cluster{"TetrixDCMotor":T4, "TetrixDCMotor":T4})
            n291 = xnode "Stop Motors"("Motors"=w1113) -> ()  [unwired: 1 in, 1 out]
          }
        }
      }
      n292 = xnode "Motors"() -> ("Motor"=w1056:T2)
      n293 = call-poly <vilib>:"PolyWait.vi"("Time (1 sec)"=sgl 0.8, "NXT/EV3"=w1027) -> ("NXT/EV3"=w1025:T7)  [unwired: 2 in]
      n294 = xnode "Move Servos"("Position 1"=u8 114, "Motors"=w1056, "NXT/EV3"=w1025) -> ("NXT/EV3"=w1049:T7)
      n295 = xnode "Motors"() -> ("Motor"=w1051:T2)
      n296 = call-poly <vilib>:"PolyWait.vi"("Time (1 sec)"=sgl 1.5, "NXT/EV3"=w1049) -> ("NXT/EV3"=w1052:T7)  [unwired: 2 in]
      n297 = xnode "Move Servos"("Position 1"=u8 40, "Motors"=w1051, "NXT/EV3"=w1052) -> ("NXT/EV3"=w1046:T7)
    }
  }
  n298 = flat-sequence {
    tunnel: w3 -> [w1260]
    tunnel: [w1249] -> w2
    frame #0 {
      w1263 = T8 2 items=["Port 1", "Port 2", "Port 3", "Port 4"] ("Port (Port 1)")
      w1272 = T8 2 items=["Port 1", "Port 2", "Port 3", "Port 4"] ("Port (Port 1)")
      n299 = xnode "Motors"() -> ("Motor"=w1282:cluster{"TetrixDCMotor":T4, "TetrixDCMotor":T4})
      n300 = call-poly <vilib>:"PolyWait.vi"("Time (1 sec)"=sgl 1.0, "NXT/EV3"=w1260) -> ("NXT/EV3"=w1259:T7)  [unwired: 2 in]
      n301 = xnode "Move Motors"("Power/Speed 2"=i8 -50, "Power/Speed 1"=i8 -50, "Motors"=w1282, "NXT/EV3"=w1259) -> ("NXT/EV3"=w1285:T7)
      n302 = call-poly <vilib>:"PolyWait.vi"("Time (1 sec)"=sgl 0.8, "NXT/EV3"=w1285) -> ("NXT/EV3"=w1284:T7)  [unwired: 2 in]
      n303 = xnode "Motors"() -> ("Motor"=w1277:cluster{"TetrixDCMotor":T4, "TetrixDCMotor":T4})
      n304 = xnode "Stop Motors"("Motors"=w1282, "NXT/EV3"=w1284) -> ("NXT/EV3"=w1275:T7)
      n305 = call-poly <vilib>:"PolyWait.vi"("Time (1 sec)"=sgl 1.0, "NXT/EV3"=w1275) -> ("NXT/EV3"=w1274:T7)  [unwired: 2 in]
      n306 = xnode "Move Motors"("Power/Speed 2"=i8 20, "Power/Speed 1"=i8 20, "Motors"=w1277, "NXT/EV3"=w1274) -> ("NXT/EV3"=w1279:T7)
      n307 = call-poly <vilib>:"PolyWait.vi"("Color (Red)"=ColorSensorColors."Black", "NXT/EV3"=w1279, "Port (Port 1)"=w1272) -> ("NXT/EV3"=w1278:T7)  [unwired: 1 in]
      n308 = xnode "Motors"() -> ("Motor"=w1267:cluster{"TetrixDCMotor":T4, "TetrixDCMotor":T4})
      n309 = xnode "Stop Motors"("Motors"=w1277, "NXT/EV3"=w1278) -> ("NXT/EV3"=w1262:T7)
      n310 = call-poly <vilib>:"PolyWait.vi"("Time (1 sec)"=sgl 0.5, "NXT/EV3"=w1262) -> ("NXT/EV3"=w1265:T7)  [unwired: 2 in]
      n311 = xnode "Move Motors"("Power/Speed 2"=i8 -20, "Power/Speed 1"=i8 -20, "Motors"=w1267, "NXT/EV3"=w1265) -> ("NXT/EV3"=w1269:T7)
      n312 = call-poly <vilib>:"PolyWait.vi"("Color (Red)"=ColorSensorColors."Black", "NXT/EV3"=w1269, "Port (Port 1)"=w1263) -> ("NXT/EV3"=w1268:T7)  [unwired: 1 in]
      n313 = xnode "Motors"() -> ("Motor"=w1253:cluster{"TetrixDCMotor":T4, "TetrixDCMotor":T4})
      n314 = xnode "Stop Motors"("Motors"=w1267, "NXT/EV3"=w1268) -> ("NXT/EV3"=w1251:T7)
      n315 = call-poly <vilib>:"PolyWait.vi"("Time (1 sec)"=sgl 0.5, "NXT/EV3"=w1251) -> ("NXT/EV3"=w1250:T7)  [unwired: 2 in]
      n316 = xnode "Move Motors"("Power/Speed 2"=i8 -5, "Power/Speed 1"=i8 -5, "Motors"=w1253, "NXT/EV3"=w1250) -> ("NXT/EV3"=w1256:T7)
      n317 = call-poly <vilib>:"PolyWait.vi"("Time (1 sec)"=sgl 1.0, "NXT/EV3"=w1256) -> ("NXT/EV3"=w1255:T7)  [unwired: 2 in]
      n318 = xnode "Stop Motors"("Motors"=w1253, "NXT/EV3"=w1255) -> ("NXT/EV3"=w1249:T7)
    }
  }
  n319 = flat-sequence {
    tunnel: [w1355] -> w1
    tunnel: w2 -> [w1344]
    frame #0 {
      w1370 = T8 1 items=["Port 1", "Port 2", "Port 3", "Port 4"] ("Port (Port 1)")
      w1387 = T8 1 items=["Port 1", "Port 2", "Port 3", "Port 4"] ("Port (Port 1)")
      n320 = xnode "Motors"() -> ("Motor"=w1354:T6)
      n321 = call-poly <vilib>:"PolyWait.vi"("Time (1 sec)"=sgl 1.0, "NXT/EV3"=w1344) -> ("NXT/EV3"=w1346:T7)  [unwired: 2 in]
      n322 = xnode "Move Servos"("Position 6"=u8 8, "Position 5"=u8 237, "Position 4"=u8 40, "Position 3"=u8 7, "Position 2"=u8 0, "Position 1"=u8 220, "Motors"=w1354, "NXT/EV3"=w1346) -> ("NXT/EV3"=w1345:T7)
      n323 = xnode "Motors"() -> ("Motor"=w1400:cluster{"TetrixDCMotor":T4, "TetrixDCMotor":T4})
      n324 = call-poly <vilib>:"PolyWait.vi"("Time (1 sec)"=sgl 1.0, "NXT/EV3"=w1345) -> ("NXT/EV3"=w1356:T7)  [unwired: 2 in]
      n325 = xnode "Move Motors"("Power/Speed 2"=i8 50, "Power/Speed 1"=i8 50, "Motors"=w1400, "NXT/EV3"=w1356) -> ("NXT/EV3"=w1403:T7)
      n326 = call-poly <vilib>:"PolyWait.vi"("Centimeters (40)"=sgl 8.0, "NXT/EV3"=w1403, "Port (Port 1)"=w1387) -> ("NXT/EV3"=w1401:T7)  [unwired: 1 in]
      n327 = xnode "Motors"() -> ("Motor"=w1367:cluster{"TetrixDCMotor":T4, "TetrixDCMotor":T4})
      n328 = xnode "Stop Motors"("Motors"=w1400, "NXT/EV3"=w1401) -> ("NXT/EV3"=w1376:T7)
      n329 = call-poly <vilib>:"PolyWait.vi"("Time (1 sec)"=sgl 1.0, "NXT/EV3"=w1376) -> ("NXT/EV3"=w1359:T7)  [unwired: 2 in]
      n330 = xnode "Move Motors"("Power/Speed 2"=i8 -5, "Power/Speed 1"=i8 -5, "Motors"=w1367, "NXT/EV3"=w1359) -> ("NXT/EV3"=w1373:T7)
      n331 = call-poly <vilib>:"PolyWait.vi"("Centimeters (50)"=sgl 6.0, "NXT/EV3"=w1373, "Port (Port 1)"=w1370) -> ("NXT/EV3"=w1371:T7)  [unwired: 1 in]
      n332 = xnode "Motors"() -> ("Motor"=w1361:cluster{"TetrixDCMotor":T4, "TetrixDCMotor":T4})
      n333 = xnode "Stop Motors"("Motors"=w1367, "NXT/EV3"=w1371) -> ("NXT/EV3"=w1365:T7)
      n334 = call-poly <vilib>:"PolyWait.vi"("Time (1 sec)"=sgl 1.0, "NXT/EV3"=w1365) -> ("NXT/EV3"=w1364:T7)  [unwired: 2 in]
      n335 = xnode "Move Motors"("Power/Speed 2"=i8 5, "Power/Speed 1"=i8 5, "Motors"=w1361, "NXT/EV3"=w1364) -> ("NXT/EV3"=w1363:T7)
      n336 = call-poly <vilib>:"PolyWait.vi"("Time (1 sec)"=sgl 1.0, "NXT/EV3"=w1363) -> ("NXT/EV3"=w1362:T7)  [unwired: 2 in]
      n337 = xnode "Motors"() -> ("Motor"=w1396:T4)
      n338 = xnode "Motors"() -> ("Motor"=w1392:T4)
      n339 = xnode "Stop Motors"("Motors"=w1361, "NXT/EV3"=w1362) -> ("NXT/EV3"=w1358:T7)
      n340 = call-poly <vilib>:"PolyWait.vi"("Time (1 sec)"=sgl 1.5, "NXT/EV3"=w1358) -> ("NXT/EV3"=w1390:T7)  [unwired: 2 in]
      n341 = xnode "Move Motors"("Power/Speed 1"=i8 5, "Motors"=w1396, "NXT/EV3"=w1390) -> ("NXT/EV3"=w1398:T7)
      n342 = xnode "Move Motors"("Power/Speed 1"=i8 5, "Motors"=w1392, "NXT/EV3"=w1390) -> ("NXT/EV3"=w1393:T7)
      n343 = xnode "Motors"() -> ("Sensor"=w1389:T8)
      n344 = xnode "Motors"() -> ("Sensor"=w1388:T8)
      n345 = call-poly <vilib>:"PolyWait.vi"("NXT/EV3"=w1398, "Port (Port 1)"=w1388) -> ("NXT/EV3"=w1397:T7)  [unwired: 2 in]
      n346 = call-poly <vilib>:"PolyWait.vi"("NXT/EV3"=w1393, "Port (Port 1)"=w1389) -> ("NXT/EV3"=w1391:T7)  [unwired: 2 in]
      n347 = xnode "Motors"() -> ("Motor"=w1384:cluster{"TetrixDCMotor":T4, "TetrixDCMotor":T4})
      n348 = xnode "Stop Motors"("Motors"=w1396, "NXT/EV3"=w1397) -> ()  [unwired: 1 out]
      n349 = xnode "Stop Motors"("Motors"=w1392, "NXT/EV3"=w1391) -> ("NXT/EV3"=w1386:T7)
      n350 = call-poly <vilib>:"PolyWait.vi"("Time (1 sec)"=sgl 2.0, "NXT/EV3"=w1386) -> ("NXT/EV3"=w1382:T7)  [unwired: 2 in]
      n351 = xnode "Move Motors"("Power/Speed 2"=i8 -5, "Power/Speed 1"=i8 -5, "Motors"=w1384, "NXT/EV3"=w1382) -> ("NXT/EV3"=w1379:T7)
      n352 = call-poly <vilib>:"PolyWait.vi"("Time (1 sec)"=sgl 0.2, "NXT/EV3"=w1379) -> ("NXT/EV3"=w1378:T7)  [unwired: 2 in]
      n353 = xnode "Stop Motors"("Motors"=w1384, "NXT/EV3"=w1378) -> ("NXT/EV3"=w1355:T7)
    }
  }
  n354 = flat-sequence {
    tunnel: w1 -> [w1504]
    frame #0 {
      w1507 = T8 2 items=["Port 1", "Port 2", "Port 3", "Port 4"] ("Port (Port 1)")
      w1535 = T8 2 items=["Port 1", "Port 2", "Port 3", "Port 4"] ("Port (Port 1)")
      n355 = xnode "Motors"() -> ("Motor"=w1554:cluster{"TetrixDCMotor":T4, "TetrixDCMotor":T4})
      n356 = call-poly <vilib>:"PolyWait.vi"("Time (1 sec)"=sgl 1.5, "NXT/EV3"=w1504) -> ("NXT/EV3"=w1503:T7)  [unwired: 2 in]
      n357 = xnode "Move Motors"("Power/Speed 2"=i8 -100, "Power/Speed 1"=i8 -100, "Motors"=w1554, "NXT/EV3"=w1503) -> ("NXT/EV3"=w1557:T7)
      n358 = call-poly <vilib>:"PolyWait.vi"("Time (1 sec)"=sgl 2.0, "NXT/EV3"=w1557) -> ("NXT/EV3"=w1555:T7)  [unwired: 2 in]
      n359 = xnode "Motors"() -> ("Motor"=w1548:cluster{"TetrixDCMotor":T4, "TetrixDCMotor":T4})
      n360 = xnode "Stop Motors"("Motors"=w1554, "NXT/EV3"=w1555) -> ("NXT/EV3"=w1546:T7)
      n361 = call-poly <vilib>:"PolyWait.vi"("Time (1 sec)"=sgl 1.5, "NXT/EV3"=w1546) -> ("NXT/EV3"=w1545:T7)  [unwired: 2 in]
      n362 = xnode "Move Motors"("Power/Speed 2"=i8 -100, "Power/Speed 1"=i8 -100, "Motors"=w1548, "NXT/EV3"=w1545) -> ("NXT/EV3"=w1551:T7)
      n363 = call-poly <vilib>:"PolyWait.vi"("Time (1 sec)"=sgl 1.0, "NXT/EV3"=w1551) -> ("NXT/EV3"=w1549:T7)  [unwired: 2 in]
      n364 = xnode "Motors"() -> ("Motor"=w1538:cluster{"TetrixDCMotor":T4, "TetrixDCMotor":T4})
      n365 = xnode "Stop Motors"("Motors"=w1548, "NXT/EV3"=w1549) -> ("NXT/EV3"=w1543:T7)
      n366 = call-poly <vilib>:"PolyWait.vi"("Time (1 sec)"=sgl 1.0, "NXT/EV3"=w1543) -> ("NXT/EV3"=w1537:T7)  [unwired: 2 in]
      n367 = xnode "Move Motors"("Power/Speed 2"=i8 -5, "Power/Speed 1"=i8 -5, "Motors"=w1538, "NXT/EV3"=w1537) -> ("NXT/EV3"=w1540:T7)
      n368 = call-poly <vilib>:"PolyWait.vi"("Color (Red)"=ColorSensorColors."Black", "NXT/EV3"=w1540, "Port (Port 1)"=w1535) -> ("NXT/EV3"=w1539:T7)  [unwired: 1 in]
      n369 = xnode "Motors"() -> ("Motor"=w1529:cluster{"TetrixDCMotor":T4, "TetrixDCMotor":T4})
      n370 = xnode "Stop Motors"("Motors"=w1538, "NXT/EV3"=w1539) -> ("NXT/EV3"=w1508:T7)
      n371 = call-poly <vilib>:"PolyWait.vi"("Time (1 sec)"=sgl 0.5, "NXT/EV3"=w1508) -> ("NXT/EV3"=w1518:T7)  [unwired: 2 in]
      n372 = xnode "Move Motors"("Power/Speed 2"=i8 5, "Power/Speed 1"=i8 5, "Motors"=w1529, "NXT/EV3"=w1518) -> ("NXT/EV3"=w1530:T7)
      n373 = call-poly <vilib>:"PolyWait.vi"("Color (Red)"=ColorSensorColors."Black", "NXT/EV3"=w1530, "Port (Port 1)"=w1507) -> ("NXT/EV3"=w1531:T7)  [unwired: 1 in]
      n374 = xnode "Motors"() -> ("Motor"=w1520:cluster{"TetrixDCMotor":T4, "TetrixDCMotor":T4})
      n375 = xnode "Stop Motors"("Motors"=w1529, "NXT/EV3"=w1531) -> ("NXT/EV3"=w1527:T7)
      n376 = call-poly <vilib>:"PolyWait.vi"("Time (1 sec)"=sgl 1.0, "NXT/EV3"=w1527) -> ("NXT/EV3"=w1524:T7)  [unwired: 2 in]
      n377 = xnode "Move Motors"("Power/Speed 2"=i8 -5, "Power/Speed 1"=i8 -5, "Motors"=w1520, "NXT/EV3"=w1524) -> ("NXT/EV3"=w1522:T7)
      n378 = call-poly <vilib>:"PolyWait.vi"("Time (1 sec)"=sgl 1.23, "NXT/EV3"=w1522) -> ("NXT/EV3"=w1521:T7)  [unwired: 2 in]
      n379 = xnode "Motors"() -> ("Motor"=w1515:T6)
      n380 = xnode "Stop Motors"("Motors"=w1520, "NXT/EV3"=w1521) -> ("NXT/EV3"=w1517:T7)
      n381 = call-poly <vilib>:"PolyWait.vi"("Time (1 sec)"=sgl 1.0, "NXT/EV3"=w1517) -> ("NXT/EV3"=w1509:T7)  [unwired: 2 in]
      n382 = xnode "Move Servos"("Position 6"=u8 28, "Position 5"=u8 80, "Position 4"=u8 40, "Position 3"=u8 7, "Position 2"=u8 0, "Position 1"=u8 230, "Motors"=w1515, "NXT/EV3"=w1509) -> ()  [unwired: 1 out]
    }
  }
